vi "cdex_Position PID.vi"(9 "travel speed":dbl, 10 "travel angle":dbl, 11 "travel set point":dbl) -> (2 "Output (u)":dbl)   [LabVIEW 2014]
uses:
  <vilib>/Simulation/Implementation/Shared/SIMSCR Execution Mode.ctl
  <vilib>/Simulation/Scripting/Companion Diagram/SimConfigNode/SimParams.ctl
  <vilib>/Simulation/Scripting/Companion Diagram/SimConfigNode/_simSolvers.ctl
  <vilib>/Simulation/Param Hierarchy/Typedefs/SIMPH Param Control Actions.ctl
  <vilib>/Simulation/Implementation/Shared/SIM limit type.ctl
  <vilib>/Simulation/Implementation/Shared/NILVSim_ParamChanged.vi
  <vilib>/Simulation/Implementation/Shared/NILVSIM_BeginStep.vi
  <vilib>/Simulation/SignalArithmetic/Implementation/NILVSim Gain.llb/SIM Gain (scalar).vi
  <vilib>/Simulation/Nonlinear/Implementation/NILVSim Saturation.llb/SIM Saturation (scalar).vi
  <vilib>/Simulation/ContinuousLinear/Implementation/NILVSim Integrator new.llb/SIM Integrator distributor (scalar).vi
  <vilib>/Simulation/ContinuousLinear/Implementation/NILVSim Integrator new.llb/SIM Integrator collector (scalar).vi
  <vilib>/Simulation/Implementation/Shared/NILVSim_Manager.vi
  <vilib>/Utility/error.llb/Clear Errors.vi
  <vilib>/Simulation/Implementation/Shared/NILVSim_FinalizeModel.vi
  <vilib>/Simulation/Implementation/Shared/SIM Unbundle Sim Info.vi
  <vilib>/Simulation/Implementation/Shared/SIMSH Read Queue.vi
  3DHe_Global.vi
  <vilib>/Simulation/Implementation/Shared/NILVSim_Initialize.vi
  <vilib>/Simulation/Utility/Implementation/NILVSim Get Time and IsAcceptedStep.vi
  <vilib>/Simulation/Implementation/Shared/NILVSim_GetModelError.vi
  <vilib>/Simulation/Implementation/Shared/SIM SimErrorHandler.vi
  <vilib>/Simulation/Implementation/Shared/SIM Bundle Sim Info.vi
  <vilib>/Simulation/Scripting/Companion Diagram/SimConfigNode/SimDog.xnode
  <vilib>/Simulation/Implementation/XNodeFramework/SimXNode/SimX.xnode
  <vilib>/Simulation/ContinuousLinear/Implementation/NILVSim Integrator new.llb/SIM Integrator (scalar).vi
  <vilib>/Simulation/Implementation/Shared/NI_SIM_Implementation.lvlib
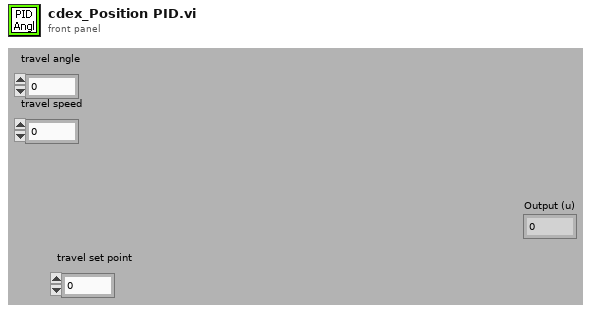
[diagram p1: front panel]
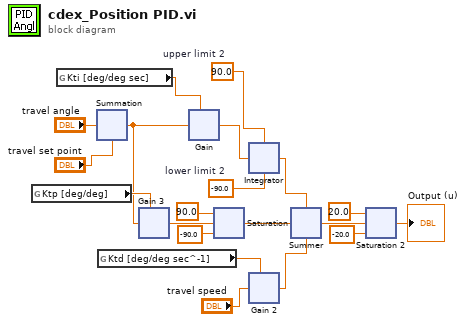
[diagram p0: block diagram]
diagram:
  w15 = -90.0  # lower limit 2
  w16 = 90.0  # upper limit 2
  n1 = global read "3DHe_Global.vi 3" "Ktp [deg/deg]"() -> (w6:dbl)
  n2 = global read "3DHe_Global.vi 2" "Kti [deg/deg sec]"() -> (w5:dbl)
  n3 = xnode ("Summation")("Operand1"="travel angle", "Operand2"="travel set point") -> ("Result"=w3:dbl)
  n4 = global read "3DHe_Global.vi" "Ktd [deg/deg sec^-1]"() -> (w4:dbl)
  n5 = xnode ("Gain 3")("gain"=w6, "input"=w3) -> ("output"=w7:dbl)  [unwired: 2 in]
  n6 = xnode ("Gain")("gain"=w5, "input"=w3) -> ("output"=w20:dbl)  [unwired: 2 in]
  n7 = xnode ("Saturation")("upper limit"=90.0, "input"=w7, "lower limit"=-90.0) -> ("output"=w8:dbl)  [unwired: 2 in]
  n8 = xnode ("Integrator")("upper limit"=w16, "input"=w20, "lower limit"=w15) -> ("output"=w19:dbl)  [unwired: 7 in, 2 out]
  n9 = xnode ("Gain 2")("gain"=w4, "input"="travel speed") -> ("output"=w17:dbl)  [unwired: 2 in]
  n10 = xnode ("Summer")("Operand1"=w19, "Operand2"=w8, "Operand3"=w17) -> ("Result"=w11:dbl)
  n11 = xnode ("Saturation 2")("upper limit"=20.0 ("upper limit 3"), "input"=w11, "lower limit"=-20.0 ("lower limit 3")) -> ("output"=→"Output (u)":dbl)  [unwired: 2 in]
